vi "FRCts20_Backend_Test_MultiGet.vi"() -> ()   [LabVIEW 2014, in "FRCts20_Backend_TestCode.lvlib"]
uses:
  FRCts20_Backend_TestCode.lvlib
  FRCts20_Backend_API/FRCts20_Backend_API_Request.ctl
  FRCts20_Backend_API/FRCts20_Backend_API_Status.ctl
  FRCts20_Backend_API/FRCts20_Backend_API_Command_Request.ctl
  FRCts20_Backend_API/FRCts20_Backend_API_Request.vi
  FRCts20_Backend_API/FRCts20_Backend_API.lvlib
panel:
  out "Time":u32
  out "Request Out":T1
  # "417 in series vs 320 for queues\n415 in parallel vs 310 for queues\n273 for searching through queue in `parallel` vs 275 in serial\n567 when searching through 400 in parallel\n550-570 for queues with 400\n420 when api is made reentrant for both\n2735-3320 for get/post combo for queues\n3000-3800 for keys"
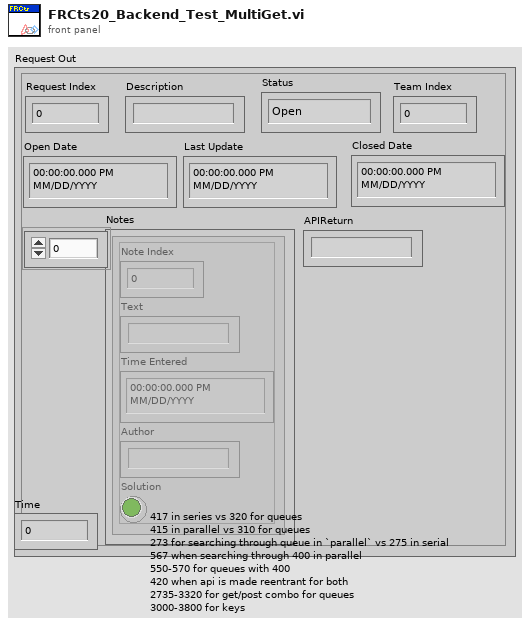
[diagram p1: front panel]
types:
  T1 = typedef "FRCts20_Backend_API.lvlib/FRCts20_Backend_API_Request.ctl" = cluster{"Request Index":u32, "Description":string, "Status":T2, "Open Date":timestamp, "Last Update":timestamp, "Closed Date":timestamp, "Notes":cluster{"Note Index":u32, "Text":string, "Time Entered":timestamp, "Author":string, "Solution":bool}[], "Team Index":u32, "APIReturn":string}
  T2 = typedef "FRCts20_Backend_API.lvlib/FRCts20_Backend_API_Status.ctl" = enum16{"Open", "In Work", "Closed"}
  T3 = typedef "FRCts20_Backend_API.lvlib/FRCts20_Backend_API_Command_Request.ctl" = string
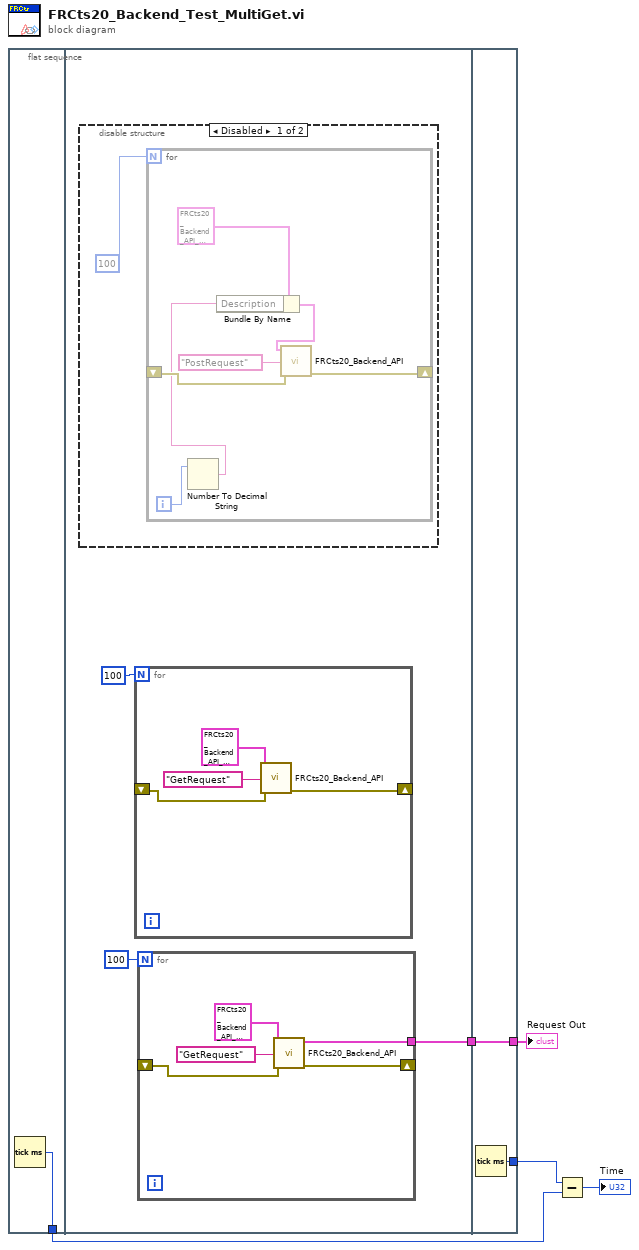
[diagram p0: block diagram]
diagram:
  n1 = flat-sequence {
    tunnel: [w6] -> w4
    tunnel: [w7] -> w3
    tunnel: [w28] -> w5
    tunnel: [w27] -> w2
    tunnel: w3 -> [w27]
    frame #0 {
      n2 = Tick Count (ms)() -> (millisecond timer value=w6:u32)
    }
    frame #1 {
      n3 = disable-structure shown="Disabled" {
        frame Disabled {
          n4 = for {
            N: 100 -> [_]
            shift-right: [w16] -> _
            shift-left: _ -> [w15]
            i -> [w12]
            n5 = Number To Decimal String(number=w12) -> (decimal integer string=w11:string)  [unwired: 1 in]
            n6 = Bundle By Name(cluster=T1 {"Request Index"=5994, "Description"="", "Status"=enum."Open", "Open Date"=timestamp(0 s since 1904-01-01), "Last Update"=timestamp(0 s since 1904-01-01), "Closed Date"=timestamp(0 s since 1904-01-01), "Notes"=[], "Team Index"=555, "APIReturn"=""} ("Request In"), "Description"=w11) -> (w13:T1)
            n7 = call-poly "FRCts20_Backend_API.vi"("error in (no error)"=w15, "Command"=T3 "PostRequest", "Request In"=w13) -> ("error out"=w16:errorcluster)  [unwired: 6 in, 2 out]
          }
        }
        frame Enabled {
        }
      }
      n8 = for {
        N: 100 -> [_]
        shift-right: [w24] -> _
        shift-left: _ -> [w23]
        n9 = call-poly "FRCts20_Backend_API.vi"("error in (no error)"=w23, "Command"=T3 "GetRequest", "Request In"=T1 {"Request Index"=5994, "Description"="", "Status"=enum."Open", "Open Date"=timestamp(0 s since 1904-01-01), "Last Update"=timestamp(0 s since 1904-01-01), "Closed Date"=timestamp(0 s since 1904-01-01), "Notes"=[], "Team Index"=0, "APIReturn"=""}) -> ("error out"=w24:errorcluster)  [unwired: 6 in, 2 out]
      }
      n10 = for {
        N: 100 -> [_]
        shift-right: [w20] -> _
        shift-left: _ -> [w19]
        tunnel: [w18] -> w7
        n11 = call-poly "FRCts20_Backend_API.vi"("error in (no error)"=w19, "Command"=T3 "GetRequest", "Request In"=T1 {"Request Index"=5994, "Description"="", "Status"=enum."Open", "Open Date"=timestamp(0 s since 1904-01-01), "Last Update"=timestamp(0 s since 1904-01-01), "Closed Date"=timestamp(0 s since 1904-01-01), "Notes"=[], "Team Index"=0, "APIReturn"=""}) -> ("error out"=w20:errorcluster, "Request Out"=w18:T1)  [unwired: 6 in, 1 out]
      }
    }
    frame #2 {
      n12 = Tick Count (ms)() -> (millisecond timer value=w28:u32)
    }
  }
  n13 = Subtract(x=w5, y=w4) -> (x-y=→"Time":u32)
  "Request Out" <- w2
